vi "Create Starter Kit 2.0 Steering Frame.vi"(8 "error in (no error)":errorcluster) -> (0 "error out":errorcluster, 3 "starter kit differential steering frame":refnum<class "NI_Robotics_Differential Steering Frame.lvclass">)   [LabVIEW 2017, in "NI_Robotics_Starter Kit Host_2.0.lvlib"]
doc: "Generates a steering frame object for the Starter Kit 2.0 robot. You can use the steering frame object with the Steering VIs to implement steering for the Starter Kit robot."
uses:
  <vilib>/robotics/Starter Kit/2.0/NI_Robotics_Starter Kit Host_2.0.lvlib
  <vilib>/robotics/Steering/Differential Steering Frame/NI_Robotics_Differential Steering Frame.lvclass
  <vilib>/robotics/Steering/Wheel/Wheel Parameters.ctl
  <vilib>/robotics/Steering/Wheel/Rotation Direction.ctl
  <vilib>/robotics/Steering/Differential Steering Frame/Create Differential Steering Frame.vi
  <vilib>/robotics/Steering/Fixed Wheel/Create Fixed Wheel.vi
  <vilib>/robotics/Steering/Wheel/NI_Robotics_Wheel.lvclass
  <vilib>/robotics/Steering/Steering Frame/NI_Robotics_Steering Frame.lvclass
  <vilib>/robotics/Steering/Fixed Wheel/NI_Robotics_Fixed Wheel.lvclass
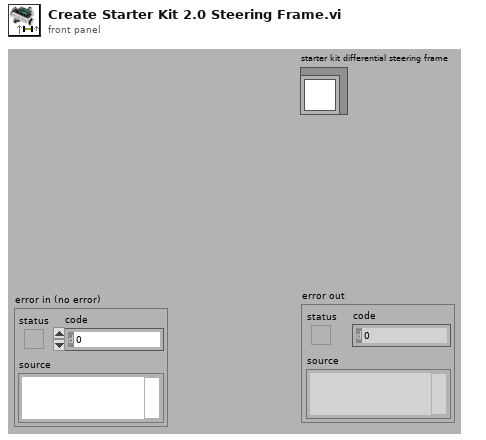
[diagram p1: front panel]
types:
  T1 = typedef "NI_Robotics_Wheel.lvclass/Wheel Parameters.ctl" = cluster{"wheel radius":dbl, "gear ratio":dbl, "forward rotation direction":T2}
  T2 = typedef "NI_Robotics_Wheel.lvclass/Rotation Direction.ctl" = u16
  T3 = cluster{"fixed wheel out":refnum<class "NI_Robotics_Fixed Wheel.lvclass">, "fixed wheel out":refnum<class "NI_Robotics_Fixed Wheel.lvclass">}
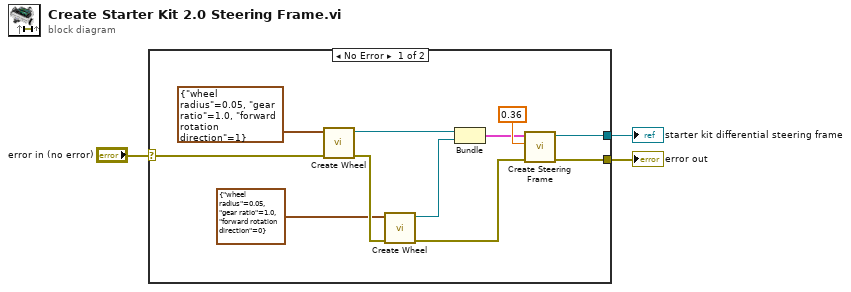
[diagram p0: block diagram]
diagram:
  n1 = case shown="No Error" "error in (no error)" {
    selector: "error in (no error)" -> [w5 w15]
    tunnel: [w7 w15] -> w2
    tunnel: [w6 _] -> w3
    frame No Error {
      n2 = call-poly <vilib>:"Create Wheel.vi"("error in (no error)"=w5, "wheel parameters"=T1 {"wheel radius"=0.05, "gear ratio"=1.0, "forward rotation direction"=1}) -> ("error out"=w11:errorcluster, "fixed wheel out"=w8:refnum<class "NI_Robotics_Fixed Wheel.lvclass">)  [unwired: 8 in]
      n3 = call-poly <vilib>:"Create Wheel.vi"("error in (no error)"=w11, "wheel parameters"=T1 {"wheel radius"=0.05, "gear ratio"=1.0, "forward rotation direction"=0}) -> ("error out"=w12:errorcluster, "fixed wheel out"=w9:refnum<class "NI_Robotics_Fixed Wheel.lvclass">)  [unwired: 8 in]
      n4 = Bundle("fixed wheel out"=w8, "fixed wheel out"=w9) -> (w10:T3)  [unwired: 1 in]
      n5 = call-poly <vilib>:"Create Steering Frame.vi"("error in (no error)"=w12, "wheel separation"=0.36, "wheels"=w10) -> ("error out"=w7:errorcluster, "differential steering frame out"=w6:refnum<class "NI_Robotics_Differential Steering Frame.lvclass">)  [unwired: 7 in]
    }
    frame Error {
    }
  }
  "starter kit differential steering frame" <- w3
  "error out" <- w2
